vi "Restart LV Dialog.vi"() -> ()   [LabVIEW 2020]
panel:
  in  "Ok":bool
  # "You must restart LabVIEW after completing this installation to enable LINX features."
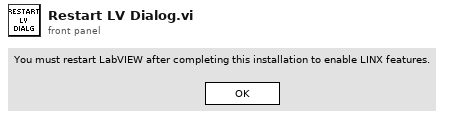
[diagram p1: front panel]
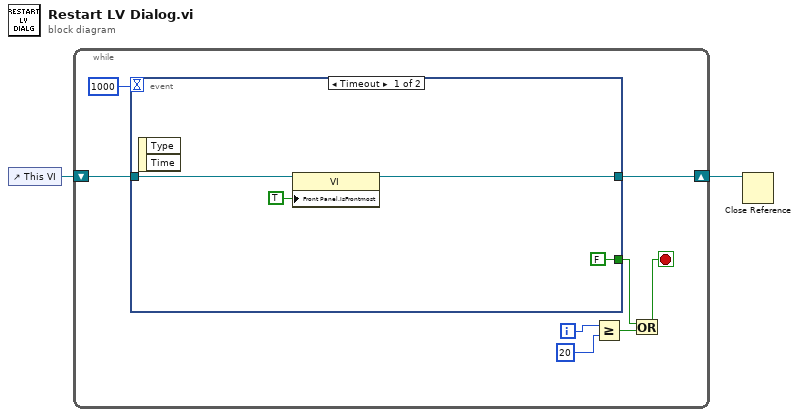
[diagram p0: block diagram]
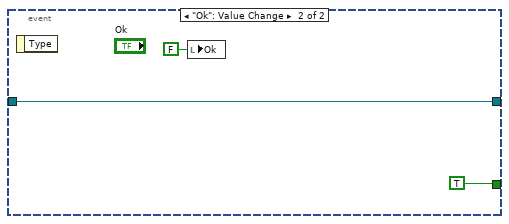
[diagram p2: hidden frame]
diagram:
  n1 = control-ref of="This VI"() -> (w1:refnum<vi>)
  n2 = while {
    shift-right: [w9] -> w2
    shift-left: w1 -> [w8]
    i -> [w5]
    stop <- w3 stop-if-true
    n3 = event shown="[0] Timeout" {
      selector: _ -> [_ _]
      dyn-events: _ -> [_ _]
      timeout: 1000 -> [_ _]
      tunnel: [FALSE ("Ok") TRUE ("Ok")] -> w4
      tunnel: [w11 w15] -> w9
      tunnel: w8 -> [w12 w15]
      event Timeout {
        n4 = event-data() -> ()  [unwired: 1 in, 2 out]
        n5 = property class="VI"(reference=w12, "Front Panel.IsFrontmost"=TRUE ("Front Panel Window:Is Frontmost")) -> (reference out=w11:refnum<vi>)  [unwired: 1 in, 1 out]
      }
      event "Ok": Value Change {
        n6 = event-data() -> ()  [unwired: 1 in, 1 out]
        n7 = local write "Ok"(FALSE ("Ok")) -> ()
      }
    }
    n8 = Greater Or Equal?(x=w5, y=20 ("x")) -> (x >= y?=w7:bool)
    n9 = Or(x=w4, y=w7) -> (x .or. y?=w3:bool)
  }
  n10 = Close Reference(reference=w2) -> ()  [unwired: 1 in, 1 out]
